vi "Get Batch Control Values.vi"(8 "error in (no error)":errorcluster, 10 "Control Names":string[](array[string]), 11 "Rename in":refnum<class "Rename.lvclass">) -> (0 "error out":errorcluster, 2 "Values":variant[](array[variant]), 3 "Rename out":refnum<class "Rename.lvclass">)   [LabVIEW 2015, in "Generic Module Library.lvlib" / "Template G_Module.lvlib" / "Rename.lvclass"]
uses:
  Rename.lvclass
  Private API/Module Control Manager/Control_Mgr_Class/Controls_Mgr.lvclass
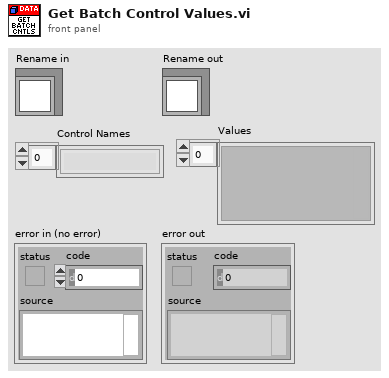
[diagram p1: front panel]
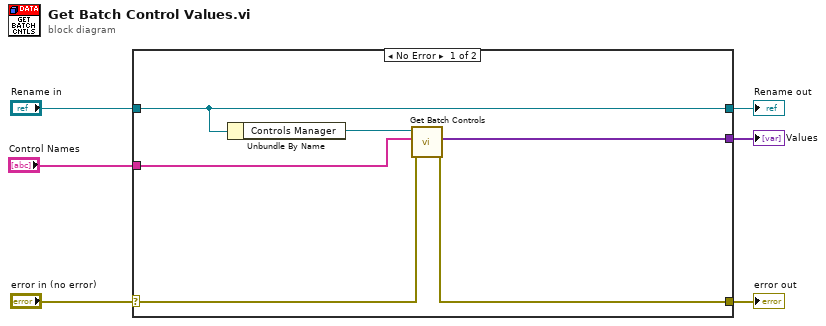
[diagram p0: block diagram]
diagram:
  n1 = case shown="No Error" "error in (no error)" {
    selector: "error in (no error)" -> [w10 w14]
    tunnel: [w9 w14] -> w5
    tunnel: [w12 w13] -> w3
    tunnel: "Rename in" -> [w12 w13]
    tunnel: "Control Names" -> [w8 _]
    tunnel: [w7 _] -> w1
    frame No Error {
      n2 = Unbundle By Name(w12) -> ("Controls Manager"=w11:refnum<class "Controls_Mgr.lvclass">)
      n3 = call "Get Batch Controls.vi"("error in (no error)"=w10, "Control Names"=w8, "Controls_Mgr in"=w11) -> ("error out"=w9:errorcluster, "Values"=w7:variant[])  [unwired: 6 in, 1 out]
    }
    frame Error {
    }
  }
  "error out" <- w5
  "Rename out" <- w3
  "Values" <- w1
